vi "Keithley 2000 DMM read DCV.vi"(2 "error in (no error)":errorcluster, 3 "Kethley 2001 address":i16=1) -> (0 "Reading":dbl format="%.2e", 1 "error out":errorcluster)   [LabVIEW 2013]
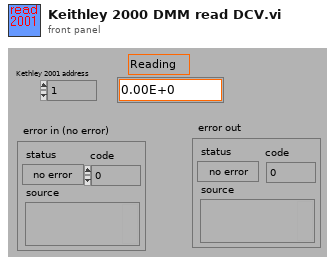
[diagram p1: front panel]
types:
  T1 = cluster{"error":bool, "code":i32, "source":string}
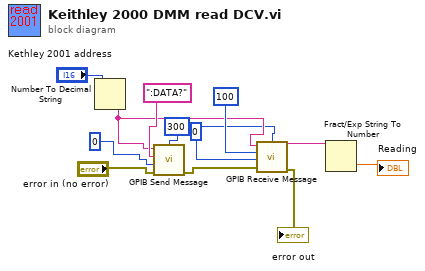
[diagram p0: block diagram]
diagram:
  w1 = 300
  n1 = Number To Decimal String(number="Kethley 2001 address") -> (decimal integer string=w5:string)  [unwired: 1 in]
  n2 = call "GPIB Send Message.vi"("timeout ms"=w1, "address string"=w5, "write buffer"=":DATA?", "write mode (set END:0)"=0, "error in"="error in (no error)") -> ("error out"=w2:T1)  [unwired: 2 in, 2 out]
  n3 = call "GPIB Receive Message.vi"("timeout ms"=w1, "address string"=w5, "byte count"=100, "read mode"=0, "error in"=w2) -> ("read buffer"=w7:string, "error out"=→"error out":T1)  [unwired: 2 in, 1 out]
  n4 = Fract/Exp String To Number(string=w7) -> (number=→"Reading":dbl)  [unwired: 3 in, 1 out]
